vi "SPC_save_sdtfile_from_databuffer.vi"(5 "SdtInfo":T1={"buf_size_x"=2, "buf_size_y"=2, "img_size_x"=2, "img_size_y"=2, "module_no"=2, "module_type"=2, "adc_resolution"=2, "is_zipped"=2, "routing_channel_num"=2, "log_mode"=2, "info_author"="", "info_company"="", "info_content"="", "serial_no"="", "logfile"=""}, 6 "SDTFilename":path, 7 "SPCdata In":T2={"base_adr"=896, "init"=0, "cfd_limit_low"=5.0, "cfd_limit_high"=80.0, "cfd_zc_level"=0.0, "cfd_holdoff"=5.0, "sync_zc_level"=0.0, "sync_holdoff"=4.0, "sync_threshold"=-20.0, "tac_range"=50.0, "sync_freq_div"=1, "tac_gain"=1, "tac_offset"=0.0, "tac_limit_low"=10.0, "tac_limit_high"=80.0, "adc_resolution"=10, "ext_latch_delay"=0, "collect_time"=0.01, "display_time"=1.0, "repeat_time"=10.0001, "stop_on_time"=1, "stop_on_ovfl"=1, "dither_range"=0, "count_incr"=1, "mem_bank"=0, "dead_time_comp"=1, "scan_control"=61440, "routing_mode"=0, "tac_enable_hold"=10.0, "pci_card_no"=-1, "mode"=0, "scan_size_x"=1, "scan_size_y"=1, "scan_rout_x"=1, "scan_rout_y"=1, "scan_flyback"=0, "scan_borders"=0, "scan_polarity"=0, "pixel_clock"=0, "line_compression"=1, "trigger"=0, "pixel_time"=5e-08, "ext_pixclk_div"=1, "rate_count_time"=1.0, "macro_time_clk"=0, "add_select"=0, "test_eep"=0, "adc_zoom"=0, "img_size_x"=1, "img_size_y"=1, "img_rout_x"=1, "img_rout_y"=1, "xy_gain"=1, "master_clock"=0, "adc_sample_delay"=0, "detector_type"=1, "chan_enable"=4191231, "chan_slope"=0, "chan_spec_no"=34835, "tdc_control"=0, "tdc_offset1"=0.0, "tdc_offset2"=0.0, "tdc_offset3"=0.0, "tdc_offset4"=0.0, "future_reserve1"=0, "future_reserve2"=0, "future_reserve3"=0, "future_reserve4"=0, "future_reserve5"=0, "future_reserve6"=0, "future_reserve7"=0}, 8 "Error In":errorcluster, 9 "FifoImageData":u16[](array[numeric]), 11 "DLL Path":path) -> (0 "Error Out":errorcluster, 2 "return":i32, 3 "DLL Path":path)   [LabVIEW 2019]
doc: "The procedure sends all parameters from the ‘SPCdata’ structure to the internal DLL structures of the module ‘mod_no’ and to the control registers of the SPC module ‘mod_no’.\nThe new parameter values are recalculated according to the parameter limits, hardware restrictions (e.g. DAC resolution) and the SPC module type. Furthermore, cross dependencies between different parameters are taken into account to ensure the correct hardware operation. \nThis VI also calls SPC_get_parameters after the call to SPC_set_parameters to provide the actual values after recalculation.\nIf an error occurs at a particular parameter, the procedure does not set the rest of the parameters and returns with an error code\n\ninfo@becker-hickl.com"
uses:
  SPC_Controls/SPCdata.ctl
  SPC_Controls/SdtInfo.ctl
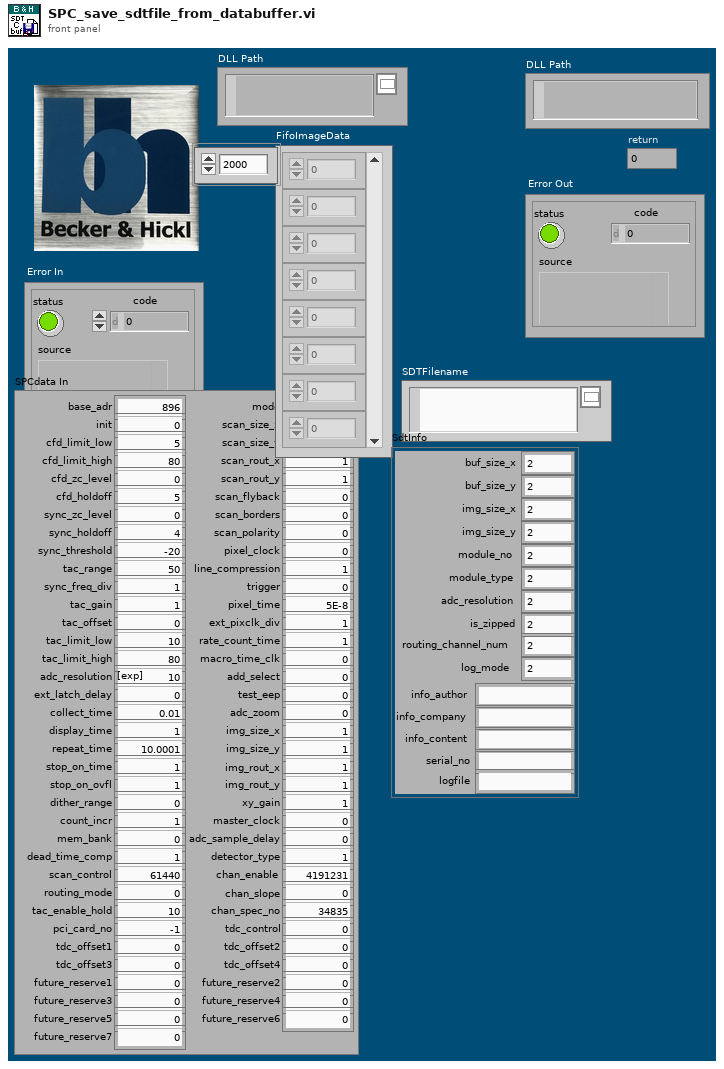
[diagram p1: front panel]
types:
  T1 = typedef "SdtInfo.ctl" = cluster{"buf_size_x":i32, "buf_size_y":i32, "img_size_x":i32, "img_size_y":i32, "module_no":i32, "module_type":i32, "adc_resolution":i32, "is_zipped":i32, "routing_channel_num":i32, "log_mode":i32, "info_author":string, "info_company":string, "info_content":string, "serial_no":string, "logfile":string}
  T2 = typedef "SPCdata.ctl" = cluster{"base_adr":u16, "init":i16, "cfd_limit_low":sgl, "cfd_limit_high":sgl, "cfd_zc_level":sgl, "cfd_holdoff":sgl, "sync_zc_level":sgl, "sync_holdoff":sgl, "sync_threshold":sgl, "tac_range":sgl, "sync_freq_div":i16, "tac_gain":i16, "tac_offset":sgl, "tac_limit_low":sgl, "tac_limit_high":sgl, "adc_resolution":i16, "ext_latch_delay":i16, "collect_time":sgl, "display_time":sgl, "repeat_time":sgl, "stop_on_time":i16, "stop_on_ovfl":i16, "dither_range":i16, "count_incr":i16, "mem_bank":i16, "dead_time_comp":i16, "scan_control":u16, "routing_mode":u16, "tac_enable_hold":sgl, "pci_card_no":i16, "mode":u16, "scan_size_x":u32, "scan_size_y":u32, "scan_rout_x":u32, "scan_rout_y":u32, "scan_flyback":u32, "scan_borders":u32, "scan_polarity":u16, "pixel_clock":u16, "line_compression":u16, "trigger":u16, "pixel_time":sgl, "ext_pixclk_div":u32, "rate_count_time":sgl, "macro_time_clk":i16, "add_select":i16, "test_eep":i16, "adc_zoom":i16, "img_size_x":u32, "img_size_y":u32, "img_rout_x":u32, "img_rout_y":u32, "xy_gain":i16, "master_clock":i16, "adc_sample_delay":i16, "detector_type":i16, "chan_enable":u32, "chan_slope":u32, "chan_spec_no":u32, "tdc_control":u32, "tdc_offset1":sgl, "tdc_offset2":sgl, "tdc_offset3":sgl, "tdc_offset4":sgl, "future_reserve1":u64, "future_reserve2":u64, "future_reserve3":u64, "future_reserve4":u64, "future_reserve5":u64, "future_reserve6":u64, "future_reserve7":u64}
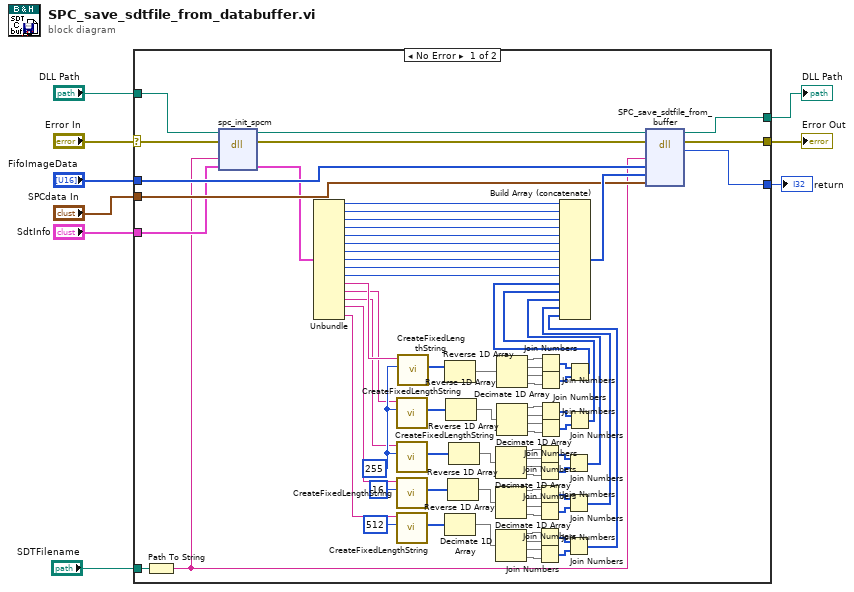
[diagram p0: block diagram]
diagram:
  n1 = case shown="No Error" "Error In" {
    selector: "Error In" -> [w61 w87]
    tunnel: "DLL Path" -> [w57 w88]
    tunnel: [w64 w87] -> w8
    tunnel: [w62 w88] -> w7
    tunnel: "SPCdata In" -> [w78 _]
    tunnel: "SDTFilename" -> [w86 _]
    tunnel: "FifoImageData" -> [w79 _]
    tunnel: "SdtInfo" -> [w59 _]
    tunnel: [w63 _] -> w1
    frame No Error {
      w71 = 255 ("RequiredStringLength")
      n2 = Path To String(path=w86) -> (string=w55:string)
      n3 = dll-call lib="C:/Users/Jannis/Documents/BH-LabVIEW-SPC-Development/Examples/FifoImage-App/spcm_64w147c19_dbg.dll" fn="spc_init_spcm"(path in=w57, error in=w61, "set_infile"=w55, "sdt_info"=w59) -> (path out=w56:path, error out=w60:errorcluster, "sdt_info"=w58:T1)  [unwired: 3 in]
      n4 = Unbundle(w58) -> ("buf_size_x"=w84:i32, "buf_size_y"=w83:i32, "img_size_x"=w82:i32, "img_size_y"=w81:i32, "module_no"=w80:i32, "module_type"=w77:i32, "adc_resolution"=w76:i32, "is_zipped"=w75:i32, "routing_channel_num"=w74:i32, "log_mode"=w73:i32, "info_author"=w72:string, "info_company"=w70:string, "info_content"=w69:string, "serial_no"=w68:string, "logfile"=w66:string)
      n5 = call "CreateFixedLengthString.vi"("RequiredStringLength"=w71, "StringIn"=w70) -> ("ByteArray"=w25:u8[])  [unwired: 8 in, 1 out]
      n6 = call "CreateFixedLengthString.vi"("RequiredStringLength"=w71, "StringIn"=w69) -> ("ByteArray"=w26:u8[])  [unwired: 8 in, 1 out]
      n7 = call "CreateFixedLengthString.vi"("RequiredStringLength"=16, "StringIn"=w68) -> ("ByteArray"=w40:u8[])  [unwired: 8 in, 1 out]
      n8 = call "CreateFixedLengthString.vi"("RequiredStringLength"=512, "StringIn"=w66) -> ("ByteArray"=w48:u8[])  [unwired: 8 in, 1 out]
      n9 = call "CreateFixedLengthString.vi"("RequiredStringLength"=w71, "StringIn"=w72) -> ("ByteArray"=w18:u8[])  [unwired: 8 in, 1 out]
      n10 = Reverse 1D Array(array=w18) -> (reversed array=w14:u8[])
      n11 = Reverse 1D Array(array=w48) -> (reversed array=w10:u8[])
      n12 = Reverse 1D Array(array=w25) -> (reversed array=w13:u8[])
      n13 = Reverse 1D Array(array=w40) -> (reversed array=w11:u8[])
      n14 = Reverse 1D Array(array=w26) -> (reversed array=w12:u8[])
      n15 = Decimate 1D Array(w12) -> (w27:u8[], w28:u8[], w29:u8[], w30:u8[])
      n16 = Decimate 1D Array(w11) -> (w41:u8[], w42:u8[], w43:u8[], w44:u8[])
      n17 = Decimate 1D Array(w10) -> (w54:u8[], w53:u8[], w52:u8[], w51:u8[])
      n18 = Decimate 1D Array(w14) -> (w19:u8[], w20:u8[], w21:u8[], w22:u8[])
      n19 = Decimate 1D Array(w13) -> (w38:u8[], w37:u8[], w36:u8[], w35:u8[])
      n20 = Join Numbers(hi=w27, lo=w28) -> ((hi.lo)=w31:u16[])
      n21 = Join Numbers(hi=w29, lo=w30) -> ((hi.lo)=w32:u16[])
      n22 = Join Numbers(hi=w41, lo=w42) -> ((hi.lo)=w45:u16[])
      n23 = Join Numbers(hi=w43, lo=w44) -> ((hi.lo)=w46:u16[])
      n24 = Join Numbers(hi=w54, lo=w53) -> ((hi.lo)=w50:u16[])
      n25 = Join Numbers(hi=w52, lo=w51) -> ((hi.lo)=w49:u16[])
      n26 = Join Numbers(hi=w19, lo=w20) -> ((hi.lo)=w23:u16[])
      n27 = Join Numbers(hi=w21, lo=w22) -> ((hi.lo)=w24:u16[])
      n28 = Join Numbers(hi=w38, lo=w37) -> ((hi.lo)=w34:u16[])
      n29 = Join Numbers(hi=w36, lo=w35) -> ((hi.lo)=w33:u16[])
      n30 = Join Numbers(hi=w31, lo=w32) -> ((hi.lo)=w15:u32[])
      n31 = Join Numbers(hi=w45, lo=w46) -> ((hi.lo)=w39:u32[])
      n32 = Join Numbers(hi=w50, lo=w49) -> ((hi.lo)=w47:u32[])
      n33 = Join Numbers(hi=w23, lo=w24) -> ((hi.lo)=w17:u32[])
      n34 = Join Numbers(hi=w34, lo=w33) -> ((hi.lo)=w16:u32[])
      n35 = Build Array (concatenate)(w84, w83, w82, w81, w80, w77, w76, w75, w74, w73, w17, w16, w15, w39, w47) -> (w85:u32[])
      n36 = dll-call lib="C:/Users/Jannis/Documents/BH-LabVIEW-SPC-Development/Examples/FifoImage-App/spcm_64w147c19_dbg.dll" fn="SPC_save_sdtfile_from_buffer"(path in=w56, error in=w60, "dest_file"=w55, "buffer"=w79, "sdt_info"=w85, "spc_data"=w78) -> (path out=w62:path, error out=w64:errorcluster, "return type"=w63:i32)  [unwired: 5 in]
    }
    frame Error {
    }
  }
  "DLL Path" <- w7
  "Error Out" <- w8
  "return" <- w1
